vi "readLasers.vi"(6 "Laser Readings In":T1, 7 "Reset Count":bool, 8 "Simple Laser 2":bool, 9 "Simple Laser 1":bool, 10 "Fancy Laser 2":bool, 11 "Fancy Laser 1":bool) -> (4 "Laser Readings":T1)   [LabVIEW 2017]
uses:
  Type Defs/allLaserReadings.ctl
  Type Defs/laserReading.ctl
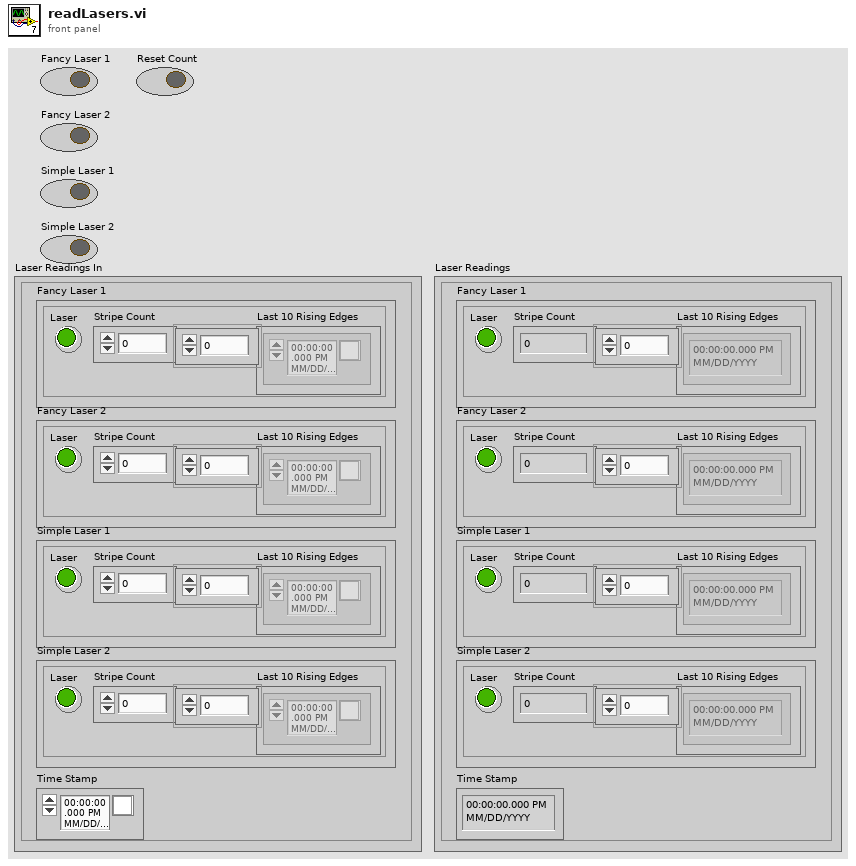
[diagram p1: front panel]
types:
  T1 = typedef "allLaserReadings.ctl" = cluster{"Fancy Laser 1":T2, "Fancy Laser 2":T2, "Simple Laser 1":T2, "Simple Laser 2":T2, "Time Stamp":timestamp}
  T2 = typedef "laserReading.ctl" = cluster{"Laser":bool, "Stripe Count":u32, "Last 10 Rising Edges":timestamp[]}
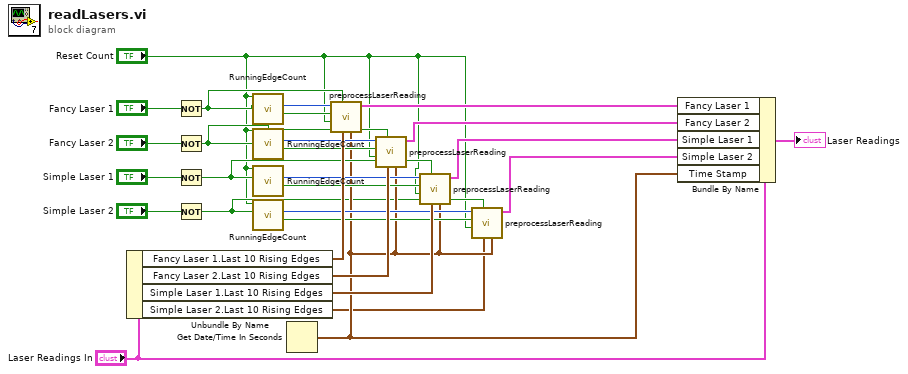
[diagram p0: block diagram]
diagram:
  n1 = Unbundle By Name("Laser Readings In") -> ("Fancy Laser 1.Last 10 Rising Edges"=w19:timestamp[], "Fancy Laser 2.Last 10 Rising Edges"=w15:timestamp[], "Simple Laser 1.Last 10 Rising Edges"=w12:timestamp[], "Simple Laser 2.Last 10 Rising Edges"=w3:timestamp[])
  n2 = Not(x="Fancy Laser 1") -> (.not. x?=w22:bool)
  n3 = Not(x="Fancy Laser 2") -> (.not. x?=w16:bool)
  n4 = Not(x="Simple Laser 1") -> (.not. x?=w11:bool)
  n5 = Not(x="Simple Laser 2") -> (.not. x?=w2:bool)
  n6 = call "RunningEdgeCount.vi"("Reset Count? (F)"="Reset Count", "Input"=w22) -> ("Rising Edge?"=w23:bool, "Count"=w24:u32)  [unwired: 8 in]
  n7 = call "RunningEdgeCount.vi"("Reset Count? (F)"="Reset Count", "Input"=w16) -> ("Rising Edge?"=w17:bool, "Count"=w18:u32)  [unwired: 8 in]
  n8 = call "RunningEdgeCount.vi"("Reset Count? (F)"="Reset Count", "Input"=w11) -> ("Rising Edge?"=w13:bool, "Count"=w14:u32)  [unwired: 8 in]
  n9 = call "RunningEdgeCount.vi"("Reset Count? (F)"="Reset Count", "Input"=w2) -> ("Rising Edge?"=w9:bool, "Count"=w10:u32)  [unwired: 8 in]
  n10 = Get Date/Time In Seconds() -> (seconds since 1Jan1904=w4:timestamp)
  n11 = call "preprocessLaserReading.vi"("Right Now"=w4, "Last 10 Rising Edges"=w19, "Laser On?"=w22, "Reset"="Reset Count", "Rising Edge?"=w23, "Count"=w24) -> ("Laser Reading"=w21:T2)  [unwired: 5 in]
  n12 = call "preprocessLaserReading.vi"("Right Now"=w4, "Last 10 Rising Edges"=w15, "Laser On?"=w16, "Reset"="Reset Count", "Rising Edge?"=w17, "Count"=w18) -> ("Laser Reading"=w8:T2)  [unwired: 5 in]
  n13 = call "preprocessLaserReading.vi"("Right Now"=w4, "Last 10 Rising Edges"=w12, "Laser On?"=w11, "Reset"="Reset Count", "Rising Edge?"=w13, "Count"=w14) -> ("Laser Reading"=w7:T2)  [unwired: 5 in]
  n14 = call "preprocessLaserReading.vi"("Right Now"=w4, "Last 10 Rising Edges"=w3, "Laser On?"=w2, "Reset"="Reset Count", "Rising Edge?"=w9, "Count"=w10) -> ("Laser Reading"=w6:T2)  [unwired: 5 in]
  n15 = Bundle By Name(cluster="Laser Readings In", "Fancy Laser 1"=w21, "Fancy Laser 2"=w8, "Simple Laser 1"=w7, "Simple Laser 2"=w6, "Time Stamp"=w4) -> (→"Laser Readings":T1)
